vi "changeBackgroundColor.vi"(8 "error in (no error)":errorcluster, 10 "Color (transparent)":u32(colorbox)=16777216, 11 "QControl_Graph in":refnum<class "QControl_Graph.lvclass">) -> (0 "error out":errorcluster, 3 "QControl_Graph out":refnum<class "QControl_Graph.lvclass">)   [LabVIEW 2017, in "QControl_Graph.lvclass"]
uses:
  QControl_Graph.lvclass
  C:/Program Files (x86)/National Instruments/LabVIEW 2017/vi.lib/QSI/QControls/QControl Classes/GraphChart/GraphChart.lvclass
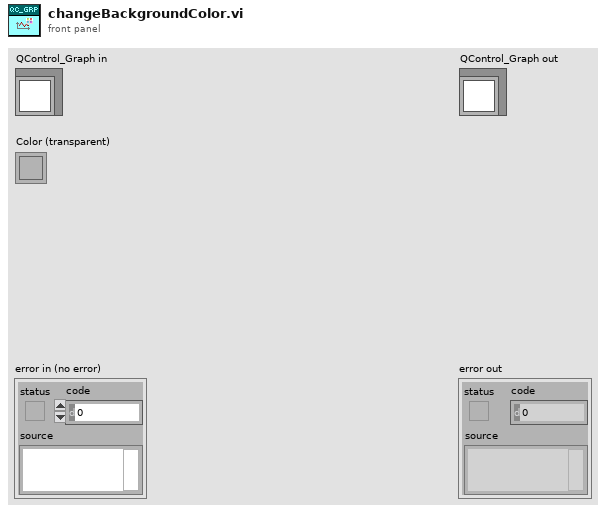
[diagram p1: front panel]
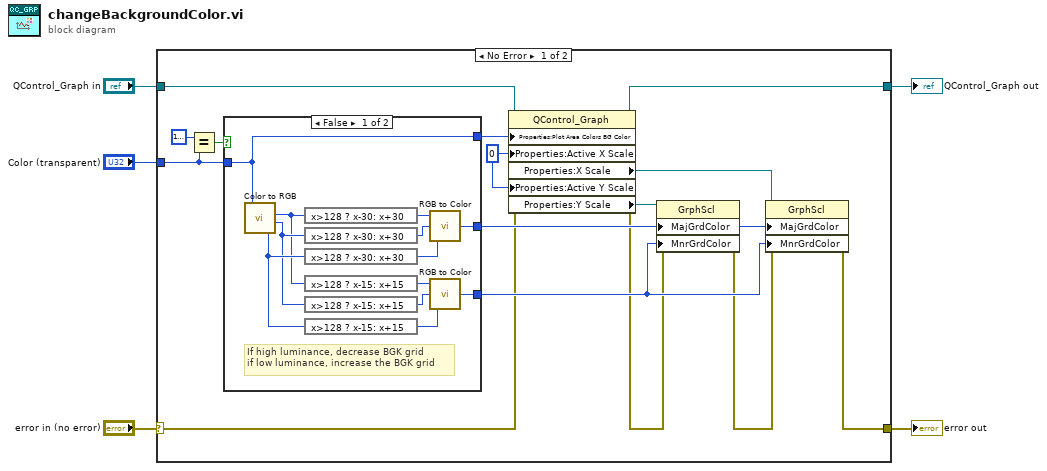
[diagram p0: block diagram]
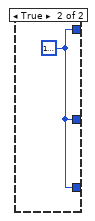
[diagram p2: hidden frame]
diagram:
  n1 = case shown="No Error" "error in (no error)" {
    selector: "error in (no error)" -> [w7 w35]
    tunnel: [w19 w35] -> w4
    tunnel: [w18 w34] -> w2
    tunnel: "QControl_Graph in" -> [w20 w34]
    tunnel: "Color (transparent)" -> [w6 _]
    frame No Error {
      w13 = 0 ("Active X Scale")
      n2 = Equal?(x=u32 16777216, y=w6) -> (x = y?=w17:bool)
      n3 = case shown="False" w17 {
        tunnel: [w32 w33] -> w10
        tunnel: [w31 w33] -> w11
        tunnel: w6 -> [w21 _]
        tunnel: [w21 w33] -> w12
        frame False {
          # "If high luminance, decrease BGK grid\nif low luminance, increase the BGK grid"
          n4 = call <vilib>:"Color to RGB.vi"("Color"=w21) -> ("R"=w22:u8, "G"=w23:u8, "B"=w24:u8)  [unwired: 1 out]
          n5 = expression code="x>128 ? x-30: x+30"(w22) -> (w25:u8)
          n6 = expression code="x>128 ? x-30: x+30"(w23) -> (w26:u8)
          n7 = expression code="x>128 ? x-30: x+30"(w24) -> (w27:u8)
          n8 = expression code="x>128 ? x-15: x+15"(w22) -> (w28:u8)
          n9 = expression code="x>128 ? x-15: x+15"(w23) -> (w29:u8)
          n10 = expression code="x>128 ? x-15: x+15"(w24) -> (w30:u8)
          n11 = call <vilib>:"RGB to Color.vi"("B"=w27, "G"=w26, "R"=w25) -> ("Color"=w31:u32)
          n12 = call <vilib>:"RGB to Color.vi"("B"=w30, "G"=w29, "R"=w28) -> ("Color"=w32:u32)
        }
        frame True {
          w33 = u32 16777216
        }
      }
      n13 = property class="QControl_Graph"(reference=w20, error in=w7, "Properties:Plot Area Colors BG Color"=w12, "Properties:Active X Scale"=w13, "Properties:Active Y Scale"=w13) -> (reference out=w18:refnum<class "QControl_Graph.lvclass">, error out=w9:errorcluster, "Properties:X Scale"=w15:refnum<vi>, "Properties:Y Scale"=w14:refnum<vi>)
      n14 = property class="GrphScl"(reference=w14, error in=w9, "MajGrdColor"=w11, "MnrGrdColor"=w10) -> (error out=w8:errorcluster)  [unwired: 1 out]
      n15 = property class="GrphScl"(reference=w15, error in=w8, "MajGrdColor"=w11, "MnrGrdColor"=w10) -> (error out=w19:errorcluster)  [unwired: 1 out]
    }
    frame Error {
    }
  }
  "error out" <- w4
  "QControl_Graph out" <- w2
